vi "RemoveWatchdog.vi"(8 "error in (no error)":errorcluster, 10 "Watchdog":refnum<data-value>, 11 "Pound in":refnum<class "Pound.lvclass">) -> (0 "error out":errorcluster, 3 "Pound out":refnum<class "Pound.lvclass">)   [LabVIEW 2017, in "Pound.lvclass"]
doc: "Remove a watchdog from the pack."
uses:
  <vilib>/NI/Software Watchdog/Pound/Pound.lvclass
  <vilib>/NI/Software Watchdog/Watchdog/Watchdog.lvclass
  <vilib>/NI/Software Watchdog/Pound/Pound.lvclass/Pound.ctl
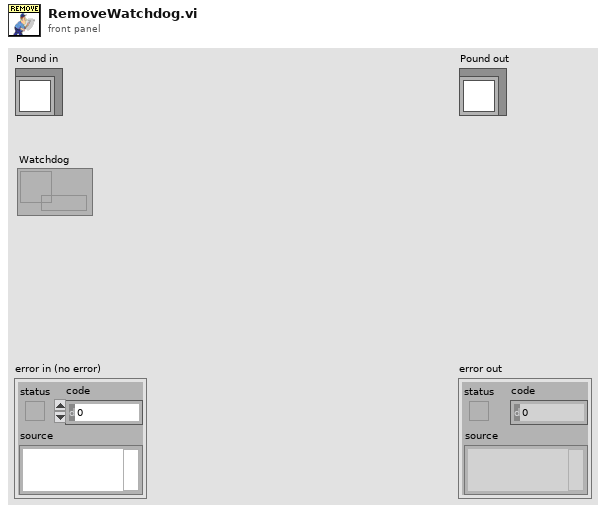
[diagram p1: front panel]
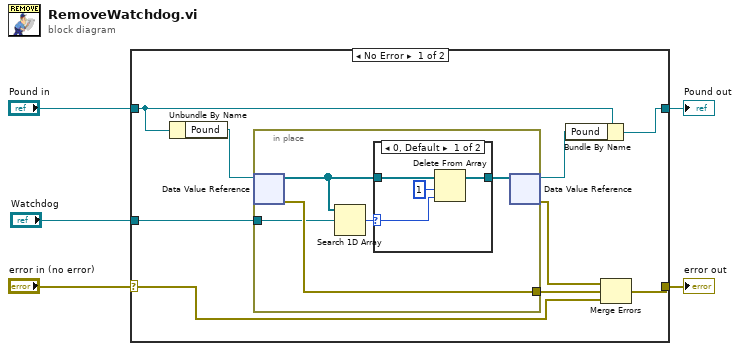
[diagram p0: block diagram]
diagram:
  n1 = case shown="No Error" "error in (no error)" {
    selector: "error in (no error)" -> [w6 w26]
    tunnel: [w7 w26] -> w4
    tunnel: [w11 w25] -> w2
    tunnel: "Pound in" -> [w12 w25]
    tunnel: "Watchdog" -> [w13 _]
    frame No Error {
      n2 = Unbundle By Name(w12) -> ("Pound"=w14:refnum<data-value>)
      n3 = in-place {
        in-place-border: w13 -> [w18]
        in-place-border: [w19] -> w8
        n4 = in-place-dvr #1(w14) -> (w17:refnum<data-value>[], w19:errorcluster)
        n5 = Search 1D Array(1D array=w17, element=w18) -> (index of element=w16:i32)  [unwired: 1 in]
        n6 = case shown="0, Default" w16 {
          selector: w16 -> [w22 _]
          tunnel: w17 -> [w21 w24]
          tunnel: [w20 w24] -> w15
          frame 0, Default {
            n7 = Delete From Array(array=w21, length=1, index=w22) -> (array with subset deleted=w20:refnum<data-value>[])  [unwired: 1 out]
          }
          frame -1 {
          }
        }
        n8 = in-place-dvr #1(w15) -> (w10:refnum<data-value>, w9:errorcluster)
      }
      n9 = Bundle By Name(cluster=w12, "Pound"=w10) -> (w11:refnum<class "Pound.lvclass">)
      n10 = Merge Errors(w9, w8, w6) -> (w7:errorcluster)
    }
    frame Error {
    }
  }
  "error out" <- w4
  "Pound out" <- w2
